vi "DB_Action-GetModuleSNExist.vi"(8 "error in":errorcluster, 9 "Name":string="1") -> (0 "error out":errorcluster={"status"=TRUE, "code"=-2147467259, "source"="ADO Connection Open.vi->DB_Action.vi->DB_Action-GetModuleConfig.vi中的Exception occured in Microsoft JET Database Engine: 找不到文件 'E:\\FCT File Share\\29_WDML\\SO-20969 MSNG\\7_Code\\3_Software\\0_DB_Action\\WDML.mdb'。"}, 1 "ID_Exist?":bool)   [LabVIEW 2015, in "Settings-Style.lvlib"]
uses:
  Settings-Style.lvlib
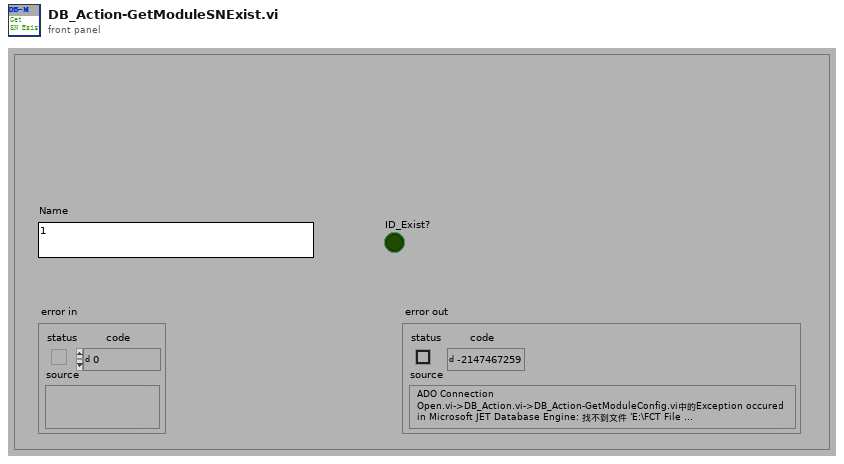
[diagram p1: front panel]
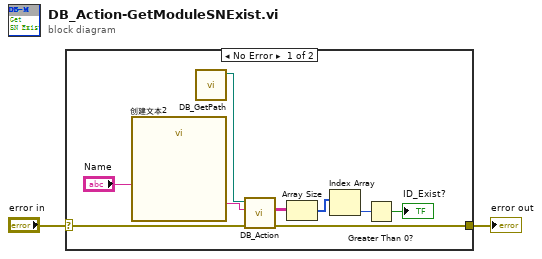
[diagram p0: block diagram]
diagram:
  n1 = case shown="No Error" "error in" {
    selector: "error in" -> [w11 w12]
    tunnel: [w9 w12] -> w2
    frame No Error {
      n2 = call "创建文本2"("Name"="Name") -> ("Result"=w10:string)  [unwired: 13 in, 1 out]
      n3 = call "DB_GetPath.vi"() -> ("appended path"=w3:path)  [unwired: 11 in]
      n4 = call "DB_Action.vi"("error in"=w11, "Command Text"=w10, "路径"=w3) -> ("error out"=w9:errorcluster, "Data"=w4:string[][])  [unwired: 7 in]
      n5 = Array Size(array=w4) -> (size(s)=w8:i32[])
      n6 = Index Array(array=w8) -> (element=w7:i32)  [unwired: 1 in]
      n7 = Greater Than 0?(x=w7) -> (x > 0?=→"ID_Exist?":bool)
    }
    frame Error {
    }
  }
  "error out" <- w2
